vi "Collide_flappy.vi"(6 "Test":bool, 7 "obs_a?":bool, 8 "error in":errorcluster, 9 "Obs D_in":refnum<vi>[](array[refnum]), 10 "Obs U_in":refnum<vi>[](array[refnum]), 11 "ball in":refnum<vi>) -> (0 "error Out":errorcluster, 2 "bump":bool)   [LabVIEW 8.6]
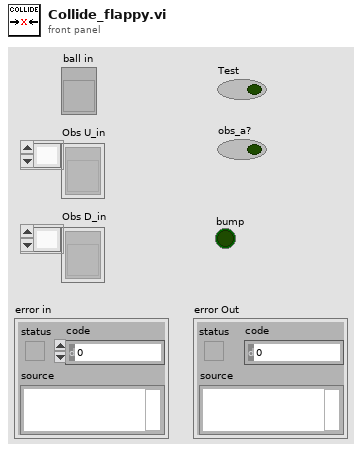
[diagram p1: front panel]
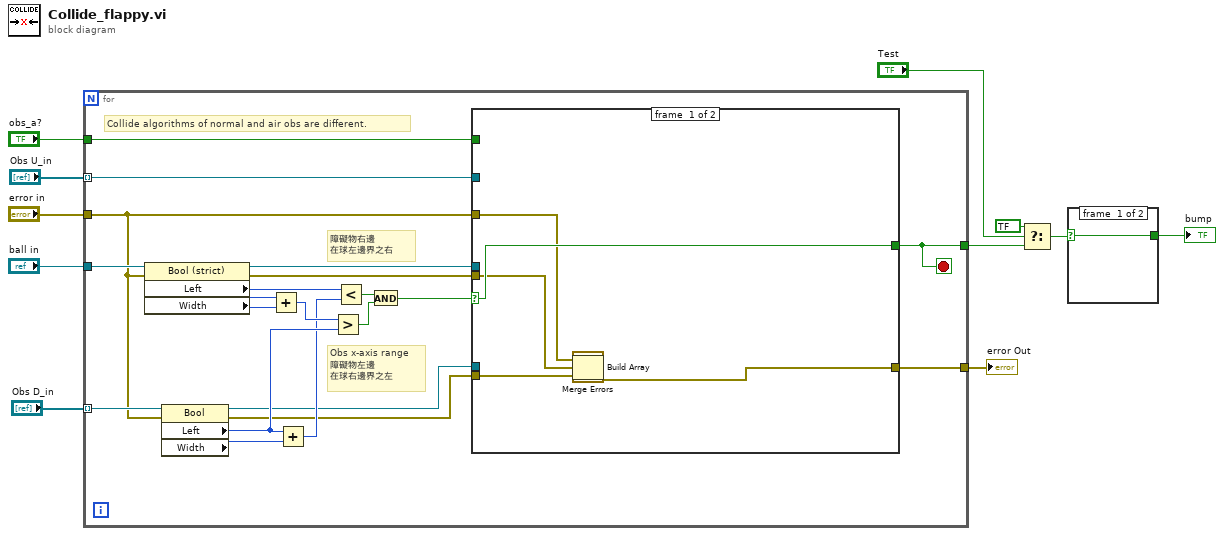
[diagram p0: block diagram]
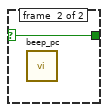
[diagram p2: hidden frame]
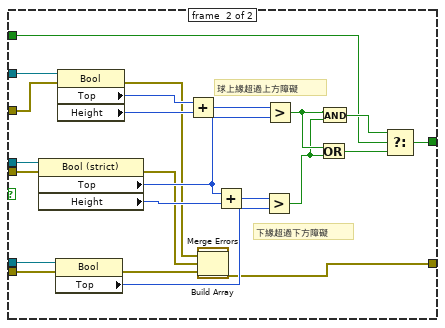
[diagram p3: hidden frame]
diagram:
  n1 = for {
    tunnel: "Obs U_in" -> [w22] mode=indexing
    tunnel: "ball in" -> [w21]
    tunnel: "Obs D_in" -> [w20] mode=indexing
    tunnel: "error in" -> [w15]
    tunnel: [w13] -> w3
    tunnel: [w14] -> w9
    tunnel: "obs_a?" -> [w12]
    stop <- w13 stop-if-true
    # "Collide algorithms of normal and air obs are different."
    # "障礙物右邊\n在球左邊界之右"
    # "Obs x-axis range\n障礙物左邊\n在球右邊界之左"
    n2 = property on="Property Node" class="Bool (strict)"(reference=w21, error in=w15) -> (reference out=w18:refnum<vi>, error out=w17:errorcluster, "Left"=w25:i32, "Width"=w26:u32)
    n3 = property on="Property Node" class="Bool"(reference=w20, error in=w15) -> (reference out=w19:refnum<vi>, error out=w16:errorcluster, "Left"=w28:i32, "Width"=w23:u32)
    n4 = Add(x=w25, y=w26) -> (x+y=w27:u32)
    n5 = Add(x=w28, y=w23) -> (x+y=w24:u32)
    n6 = Greater?(x=w27, y=w28) -> (0:w30:bool)
    n7 = Less?(x=w25, y=w24) -> (x < y?=w29:bool)
    n8 = And(x=w29, y=w30) -> (x .and. y?=w31:bool)
    n9 = case shown="True" w31 {
      selector: w31 -> [w37 _]
      tunnel: [w37 w43] -> w13
      tunnel: w22 -> [_ w56]
      tunnel: w18 -> [_ w55]
      tunnel: w19 -> [_ w54]
      tunnel: w17 -> [w34 w53]
      tunnel: w16 -> [w36 w52]
      tunnel: w15 -> [w33 w51]
      tunnel: [w35 w45] -> w14
      tunnel: w12 -> [_ w41]
      frame #0 {
        n10 = Build Array(w33, w34, w36) -> (w32:errorcluster[])
        n11 = call <vilib>:"Merge Errors.vi"("error array in"=w32) -> ("error out"=w35:errorcluster)  [unwired: 6 in]
      }
      frame #1 {
        # "球上緣超過上方障礙"
        # "下緣超過下方障礙"
        n12 = property on="Property Node" class="Bool (strict)"(reference=w55, error in=w53) -> (error out=w48:errorcluster, "Top"=w50:i32, "Height"=w59:u32)  [unwired: 1 out]
        n13 = property on="Property Node" class="Bool"(reference=w54, error in=w52) -> (error out=w47:errorcluster, "Top"=w57:i32)  [unwired: 1 out]
        n14 = property on="Property Node" class="Bool"(reference=w56, error in=w51) -> (error out=w46:errorcluster, "Top"=w60:i32, "Height"=w61:u32)  [unwired: 1 out]
        n15 = Add(x=w60, y=w61) -> (x+y=w49:u32)
        n16 = Build Array(w46, w48, w47) -> (w38:errorcluster[])
        n17 = call <vilib>:"Merge Errors.vi"("error array in"=w38) -> ("error out"=w45:errorcluster)  [unwired: 6 in]
        n18 = Add(x=w50, y=w59) -> (x+y=w58:u32)
        n19 = Greater?(x=w58, y=w57) -> (0:w39:bool)
        n20 = Greater?(x=w49, y=w50) -> (0:w40:bool)
        n21 = Or(x=w40, y=w39) -> (x .or. y?=w44:bool)
        n22 = And(x=w40, y=w39) -> (x .and. y?=w42:bool)
        n23 = Select(t=w42, s=w41, f=w44) -> (s? t:f=w43:bool)
      }
    }
  }
  "error Out" <- w9
  n24 = Select(t=bool ?, s="Test", f=w3) -> (s? t:f=w2:bool)
  n25 = case shown="True" w2 {
    selector: w2 -> [w62 w63]
    tunnel: [w62 w63] -> w1
    frame #0 {
    }
    frame #1 {
      n26 = call "beep_pc.vi"() -> ()  [unwired: 4 in, 1 out]
    }
  }
  "bump" <- w1
